vi "setCleanCount.vi"(6 "Delay between send and receive [ms]":i32=100, 8 "error in (no error)":errorcluster, 9 "mode":i32, 10 "count":i32, 11 "CCD in":refnum<class "CCD.lvclass">) -> (0 "error out":errorcluster, 1 "ID":i32, 2 "results-JSON string":string, 3 "CCD out":refnum<class "CCD.lvclass">)   [LabVIEW 2023, in "CCD.lvclass"]
doc: "Sets the number of cleans to be performed according to the specified mode setting.\n\nparameter description\nindex Integer. Used to identify which CCD to target. See ccd_list command\ncount Integer. Number of cleans.\nmode Integer. Specifies how the cleans will be performed.\n0 = Never\n1 = First Only\n2 = Between Only\n3 = Each"
uses:
  CCD.lvclass
  CCD.lvclass/CCD.ctl
  20f7d3bd-08ac-4524-9bed-df36c1da25a0.vi
  GenericDevice/GenericDevice.lvclass
  cab240a6-cbf4-4e2c-ab79-96d9c1b88265.vi
  28418afd-abcd-4dad-a3f7-ef0ce47be2ad.vi
panel:
  # "Connector Pane"
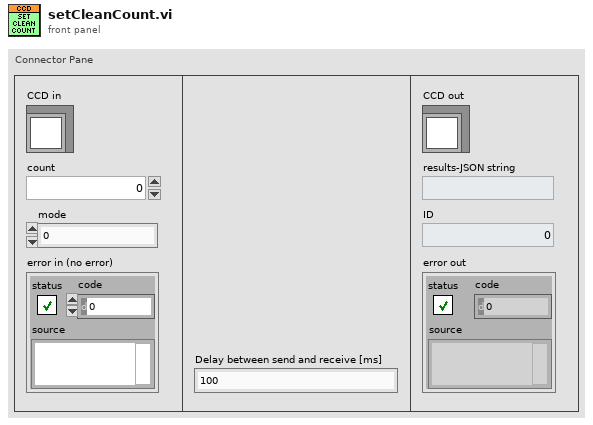
[diagram p1: front panel]
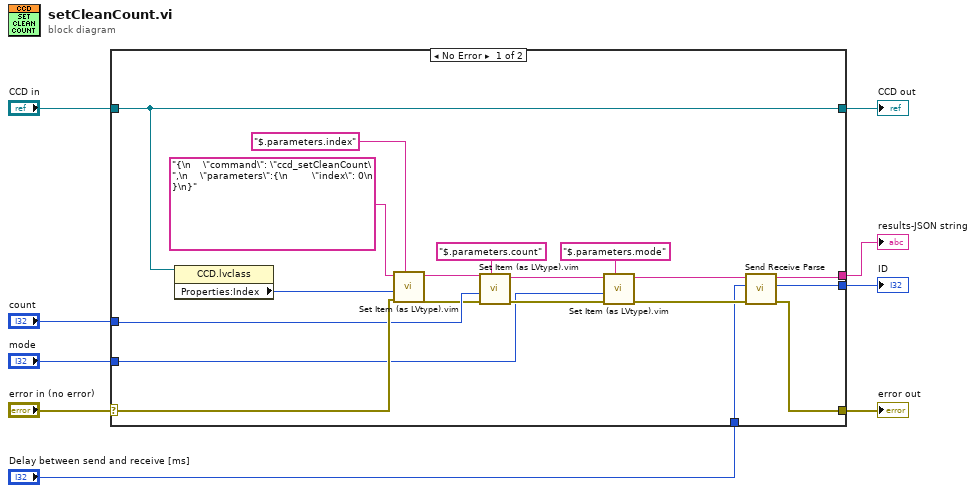
[diagram p0: block diagram]
diagram:
  n1 = case shown="No Error" "error in (no error)" {
    selector: "error in (no error)" -> [w24 w30]
    tunnel: [w19 w30] -> w8
    tunnel: [w26 w29] -> w6
    tunnel: "CCD in" -> [w26 w29]
    tunnel: "count" -> [w22 _]
    tunnel: [w18 _] -> w5
    tunnel: [w17 _] -> w4
    tunnel: "Delay between send and receive [ms]" -> [w11 _]
    tunnel: "mode" -> [w10 _]
    frame No Error {
      n2 = property class="CCD.lvclass"(reference=w26) -> ("Properties:Index"=w25:i32)  [unwired: 1 in, 2 out]
      n3 = call "Set Item (as LVtype).vim"("$Path or Item Name"="$.parameters.index", "error in (no error)"=w24, "Anything"=w25, "JSON"="{\n    \"command\": \"ccd_setCleanCount\",\n    \"parameters\":{\n        \"index\": 0\n    }\n}") -> ("error out"=w21:errorcluster, "<JSON>"=w20:string)  [unwired: 4 in, 1 out]
      n4 = call "Set Item (as LVtype).vim"("$Path or Item Name"="$.parameters.count", "error in (no error)"=w21, "Anything"=w22, "JSON"=w20) -> ("error out"=w13:errorcluster, "<JSON>"=w15:string)  [unwired: 4 in, 1 out]
      n5 = call "Set Item (as LVtype).vim"("$Path or Item Name"="$.parameters.mode", "error in (no error)"=w13, "Anything"=w10, "JSON"=w15) -> ("error out"=w12:errorcluster, "<JSON>"=w14:string)  [unwired: 4 in, 1 out]
      n6 = call "Send Receive Parse.vi"("error in"=w12, "Delay between send and receive [ms]"=w11, "<JSON>"=w14) -> ("error out"=w19:errorcluster, "ID"=w17:i32, "results-JSON string"=w18:string)  [unwired: 6 in]
    }
    frame Error {
    }
  }
  "error out" <- w8
  "CCD out" <- w6
  "results-JSON string" <- w5
  "ID" <- w4
